vi "GaussianProcessClassifier.vi"(8 "error in":errorcluster) -> (0 "error out":errorcluster, 3 "out":refnum<class "GaussianProcessClassifier.lvclass">)   [LabVIEW 2020]
doc: "Gaussian process classification (GPC) based on Laplace approximation.\n\n The implementation is based on Algorithm 3.1, 3.2, and 5.1 of\n Gaussian Processes for Machine Learning (GPML) by Rasmussen and\n Williams.\n\n Internally, the Laplace approximation is used for approximating the\n non-Gaussian posterior by a Gaussian.\n\n Currently, the implementation is restricted to using the logistic link\n function. For multi-class classification, several binary one-versus rest\n classifiers are fitted. Note that this class thus does not implement\n a true multi-class Laplace approximation.\n\n Read more in the :ref:`User Guide <gaussian_process>`.\n\n Parameters\n ----------\n kernel : kernel instance, default=None\n The kernel specifying the covariance function of the GP. If None is\n passed, the kernel \"1.0 * RBF(1.0)\" is used as default. Note that\n the kernel's hyperparameters are optimized during fitting.\n\n optimizer : 'fmin_l_bfgs_b' or callable, default='fmin_l_bfgs_b'\n Can either be one of the internally supported optimizers for optimizing\n the kernel's parameters, specified by a string, or an externally\n defined optimizer passed as a callable. If a callable is passed, it\n must have the signature::\n\n def optimizer(obj_func, initial_theta, bounds):\n # * 'obj_func' is the objective function to be maximized, which\n # takes the hyperparameters theta as parameter and an\n # optional flag eval_gradient, which determines if the\n # gradient is returned additionally to the function value\n # * 'initial_theta': the initial value for theta, which can be\n # used by local optimizers\n # * 'bounds': the bounds on the values of theta\n ....\n # Returned are the best found hyperparameters theta and\n # the corresponding value of the target function.\n return theta_opt, func_min\n\n Per default, the 'L-BFGS-B' algorithm from scipy.optimize.minimize\n is used. If None is passed, the kernel's parameters are kept fixed.\n Available internal optimizers are::\n\n 'fmin_l_bfgs_b'\n\n n_restarts_optimizer : int, default=0\n The number of restarts of the optimizer for finding the kernel's\n parameters which maximize the log-marginal likelihood. The first run\n of the optimizer is performed from the kernel's initial parameters,\n the remaining ones (if any) from thetas sampled log-uniform randomly\n from the space of allowed theta-values. If greater than 0, all bounds\n must be finite. Note that n_restarts_optimizer=0 implies that one\n run is performed.\n\n max_iter_predict : int, default=100\n The maximum number of iterations in Newton's method for approximating\n the posterior during predict. Smaller values will reduce computation\n time at the cost of worse results.\n\n warm_start : bool, default=False\n If warm-starts are enabled, the solution of the last Newton iteration\n on the Laplace approximation of the posterior mode is used as\n initialization for the next call of _posterior_mode(). This can speed\n up convergence when _posterior_mode is called several times on similar\n problems as in hyperparameter optimization. See :term:`the Glossary\n <warm_start>`.\n\n copy_X_train : bool, default=True\n If True, a persistent copy of the training data is stored in the\n object. Otherwise, just a reference to the training data is stored,\n which might cause predictions to change if the data is modified\n externally.\n\n random_state : int, RandomState instance or None, default=None\n Determines random number generation used to initialize the centers.\n Pass an int for reproducible results across multiple function calls.\n See :term: `Glossary <random_state>`.\n\n multi_class : {'one_vs_rest', 'one_vs_one'}, default='one_vs_rest'\n Specifies how multi-class classification problems are handled.\n Supported are 'one_vs_rest' and 'one_vs_one'. In 'one_vs_rest',\n one binary Gaussian process classifier is fitted for each class, which\n is trained to separate this class from the rest. In 'one_vs_one', one\n binary Gaussian process classifier is fitted for each pair of classes,\n which is trained to separate these two classes. The predictions of\n these binary predictors are combined into multi-class predictions.\n Note that 'one_vs_one' does not support predicting probability\n estimates.\n\n n_jobs : int, default=None\n The number of jobs to use for the computation: the specified\n multiclass problems are computed in parallel.\n ``None`` means 1 unless in a :obj:`joblib.parallel_backend` context.\n ``-1`` means using all processors. See :term:`Glossary <n_jobs>`\n for more details.\n\n Attributes\n ----------\n base_estimator_ : ``Estimator`` instance\n The estimator instance that defines the likelihood function\n using the observed data.\n\n kernel_ : kernel instance\n The kernel used for prediction. In case of binary classification,\n the structure of the kernel is the same as the one passed as parameter\n but with optimized hyperparameters. In case of multi-class\n classification, a CompoundKernel is returned which consists of the\n different kernels used in the one-versus-rest classifiers.\n\n log_marginal_likelihood_value_ : float\n The log-marginal-likelihood of ``self.kernel_.theta``\n\n classes_ : array-like of shape (n_classes,)\n Unique class labels.\n\n n_classes_ : int\n The number of classes in the training data\n\n \nAvailable methods:\nGet Attributes\nGet Params\nSet Params"
uses:
  Gaussian_process/GaussianProcessClassifier/GaussianProcessClassifier.lvclass
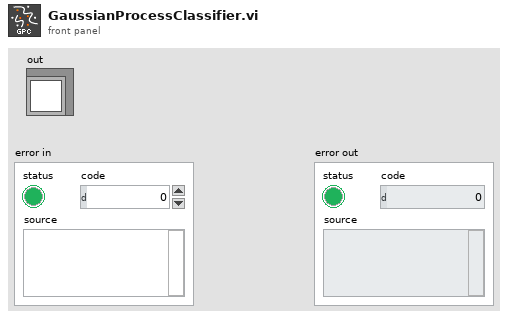
[diagram p1: front panel]
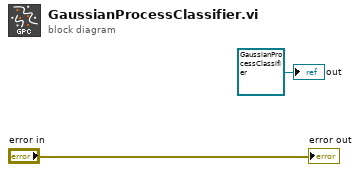
[diagram p0: block diagram]
diagram:
  "out" <- refnum<class "GaussianProcessClassifier.lvclass"> refnum ("model")
  "error out" <- "error in"
